vi "RT-test2.vi"(8 "布尔":bool, 9 "Load":bool, 10 "SimulatorConfig":T4, 11 "PatternConfig":T5 {"Max_Rate_[Hz]" format="%#_3p"}) -> (0 "EPTxPatternConfig":T1 {"Pattern"."Aux_4" format="%#_16g"; "Pattern"."Aux_3" format="%#_16g"; "Pattern"."Aux_2" format="%#_16g"; "Pattern"."Aux_1" format="%#_16g"; "Pattern"."Primary" format="%#_16g"}, 1 "Pattern Loading":bool, 2 "EPTxSimulatorConfig":T3, 3 "Sim Loading":bool, 4 "布尔 2":bool)   [LabVIEW 2020]
uses:
  <vilib>/Powertrain Controls/Device Drivers/Engine Position Tracking/EPTx/RevA/RT/Controls/Pattern Config.ctl
  <vilib>/Powertrain Controls/Device Drivers/Engine Position Tracking/EPTx/RevA/RT/Controls/Simulator Config.ctl
  <vilib>/Powertrain Controls/Device Drivers/Engine Position Tracking/EPTx/RevA/FPGA/Controls/EPTxSimulatorConfig.ctl
  <vilib>/Powertrain Controls/Device Drivers/Engine Position Tracking/EPTx/RevA/FPGA/Controls/EPTxPatternConfig.ctl
  <vilib>/Powertrain Controls/Device Drivers/Engine Position Tracking/EPTx/RevA/FPGA/Controls/Patterns.ctl
  <vilib>/Powertrain Controls/Device Drivers/Engine Position Tracking/EPTx/RevA/RT/Controls/EPTxPattern.ctl
  <vilib>/Powertrain Controls/Device Drivers/Engine Position Tracking/EPTx/RevA/RT/Controls/Pattern.ctl
  <vilib>/Powertrain Controls/Device Drivers/Engine Position Tracking/EPTx/RevA/RT/EPTx - RevA - RT.lvlib
  <vilib>/Powertrain Controls/Device Drivers/Engine Position Tracking/EPTx/RevA/FPGA/EPTx - RevA - FPGA.lvlib
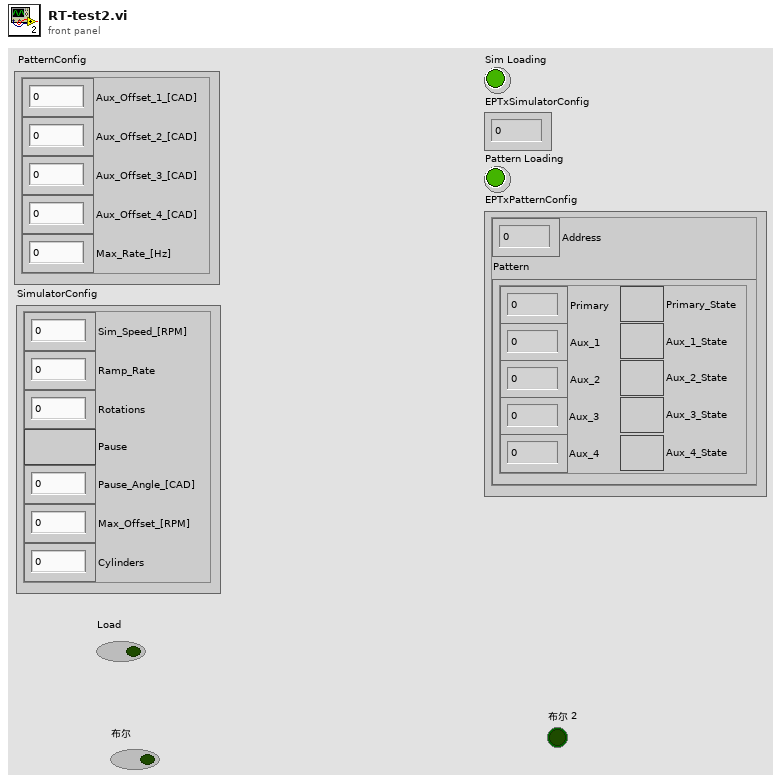
[diagram p1: front panel]
types:
  T1 = typedef "EPTx - RevA - FPGA.lvlib/EPTxPatternConfig.ctl" = cluster{"Address":fxp<+,14,14>, "Pattern":T2}
  T2 = typedef "EPTx - RevA - FPGA.lvlib/Patterns.ctl" = cluster{"Primary":fxp<+,19,12>, "Primary_State":bool, "Aux_1":fxp<+,19,12>, "Aux_1_State":bool, "Aux_2":fxp<+,19,12>, "Aux_2_State":bool, "Aux_3":fxp<+,19,12>, "Aux_3_State":bool, "Aux_4":fxp<+,19,12>, "Aux_4_State":bool}
  T3 = typedef "EPTx - RevA - FPGA.lvlib/EPTxSimulatorConfig.ctl" = u32
  T4 = typedef "EPTx - RevA - RT.lvlib/Simulator Config.ctl" = cluster{"Sim_Speed_[RPM]":sgl, "Ramp_Rate":sgl, "Rotations":u8, "Pause":bool, "Pause_Angle_[CAD]":sgl, "Max_Offset_[RPM]":sgl, "Cylinders":u8}
  T5 = typedef "EPTx - RevA - RT.lvlib/Pattern Config.ctl" = cluster{"Aux_Offset_1_[CAD]":sgl, "Aux_Offset_2_[CAD]":sgl, "Aux_Offset_3_[CAD]":sgl, "Aux_Offset_4_[CAD]":sgl, "Max_Rate_[Hz]":sgl}
  T6 = typedef "EPTx - RevA - RT.lvlib/EPTxPattern.ctl" = cluster{"Rotations":u8, "Cylinders":u8, "Primary":T7[], "Aux 1":T7[], "Aux 2":T7[], "Aux 3":T7[], "Aux 4":T7[]}
  T7 = typedef "EPTx - RevA - RT.lvlib/Pattern.ctl" = cluster{"Angle":sgl, "State":bool}
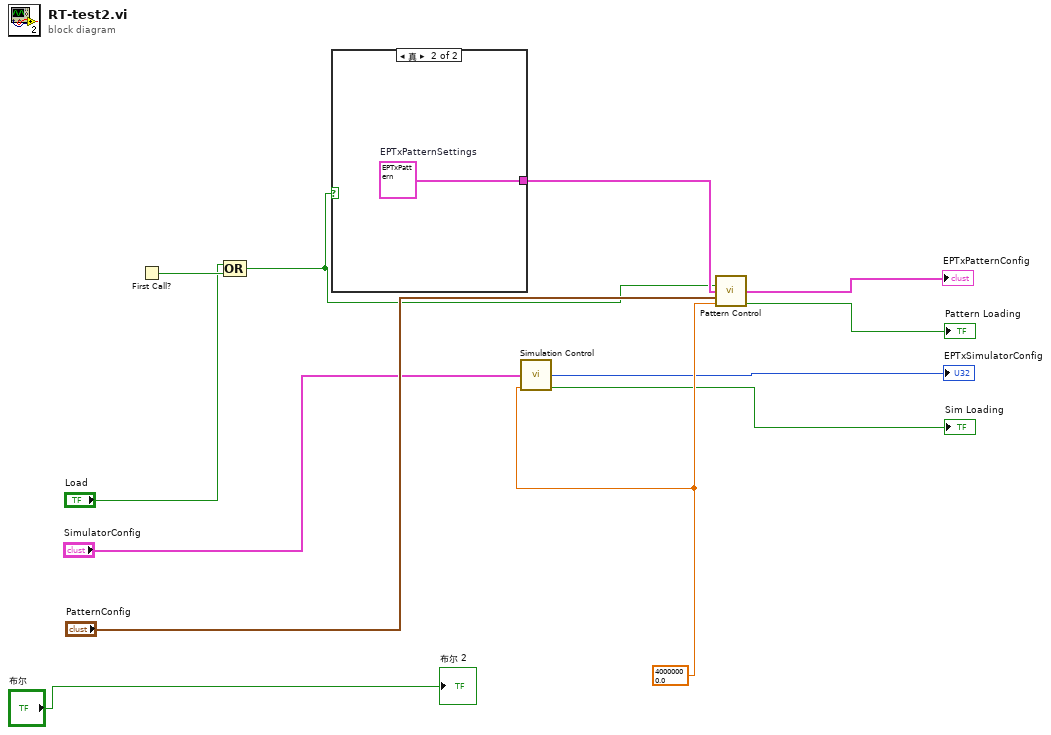
[diagram p0: block diagram]
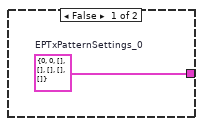
[diagram p2: hidden frame]
diagram:
  w9 = sgl 40000000.0 ("Frequency (40M) [Hz]")
  n1 = First Call?() -> (First Call?: T/F=w11:bool)
  n2 = Compound Arithmetic op=OR ("复合运算")("Load", w11) -> (w6:bool)
  n3 = case shown="真" w6 {
    tunnel: [w13 w14] -> w12
    frame False {
      w13 = T6 {"Rotations"=0, "Cylinders"=0, "Primary"=[], "Aux 1"=[], "Aux 2"=[], "Aux 3"=[], "Aux 4"=[]}  # EPTxPatternSettings_0
    }
    frame True {
      w14 = T6 {"Rotations"=2, "Cylinders"=6, "Primary"=[{"Angle"=0.0, "State"=FALSE}, {"Angle"=3.0, "State"=TRUE}, {"Angle"=6.0, "State"=FALSE}, {"Angle"=9.0, "State"=TRUE}, {"Angle"=12.0, "State"=FALSE}, {"Angle"=15.0, "State"=TRUE}, {"Angle"=18.0, "State"=FALSE}, {"Angle"=21.0, "State"=TRUE}, {"Angle"=24.0, "State"=FALSE}, {"Angle"=27.0, "State"=TRUE}, {"Angle"=30.0, "State"=FALSE}, {"Angle"=33.0, "State"=TRUE}, {"Angle"=36.0, "State"=FALSE}, {"Angle"=39.0, "State"=TRUE}, {"Angle"=42.0, "State"=FALSE}, {"Angle"=45.0, "State"=TRUE}, {"Angle"=48.0, "State"=FALSE}, {"Angle"=51.0, "State"=TRUE}, {"Angle"=54.0, "State"=FALSE}, {"Angle"=57.0, "State"=TRUE}, {"Angle"=60.0, "State"=FALSE}, {"Angle"=63.0, "State"=TRUE}, {"Angle"=66.0, "State"=FALSE}, {"Angle"=69.0, "State"=TRUE}, {"Angle"=72.0, "State"=FALSE}, {"Angle"=75.0, "State"=TRUE}, {"Angle"=78.0, "State"=FALSE}, {"Angle"=81.0, "State"=TRUE}, {"Angle"=84.0, "State"=FALSE}, {"Angle"=87.0, "State"=TRUE}, {"Angle"=90.0, "State"=FALSE}, {"Angle"=93.0, "State"=TRUE}, {"Angle"=96.0, "State"=FALSE}, {"Angle"=99.0, "State"=TRUE}, {"Angle"=102.0, "State"=FALSE}, {"Angle"=105.0, "State"=TRUE}, {"Angle"=108.0, "State"=FALSE}, {"Angle"=111.0, "State"=TRUE}, {"Angle"=114.0, "State"=FALSE}, {"Angle"=117.0, "State"=TRUE}, {"Angle"=120.0, "State"=FALSE}, {"Angle"=123.0, "State"=TRUE}, {"Angle"=126.0, "State"=FALSE}, {"Angle"=129.0, "State"=TRUE}, {"Angle"=132.0, "State"=FALSE}, {"Angle"=135.0, "State"=TRUE}, {"Angle"=138.0, "State"=FALSE}, {"Angle"=141.0, "State"=TRUE}, {"Angle"=144.0, "State"=FALSE}, {"Angle"=147.0, "State"=TRUE}, {"Angle"=150.0, "State"=FALSE}, {"Angle"=153.0, "State"=TRUE}, {"Angle"=156.0, "State"=FALSE}, {"Angle"=159.0, "State"=TRUE}, {"Angle"=162.0, "State"=FALSE}, {"Angle"=165.0, "State"=TRUE}, {"Angle"=168.0, "State"=FALSE}, {"Angle"=171.0, "State"=TRUE}, {"Angle"=174.0, "State"=FALSE}, {"Angle"=177.0, "State"=TRUE}, {"Angle"=180.0, "State"=FALSE}, {"Angle"=183.0, "State"=TRUE}, {"Angle"=186.0, "State"=FALSE}, {"Angle"=189.0, "State"=TRUE}, {"Angle"=192.0, "State"=FALSE}, {"Angle"=195.0, "State"=TRUE}, {"Angle"=198.0, "State"=FALSE}, {"Angle"=201.0, "State"=TRUE}, {"Angle"=204.0, "State"=FALSE}, {"Angle"=207.0, "State"=TRUE}, {"Angle"=210.0, "State"=FALSE}, {"Angle"=213.0, "State"=TRUE}, {"Angle"=216.0, "State"=FALSE}, {"Angle"=219.0, "State"=TRUE}, {"Angle"=222.0, "State"=FALSE}, {"Angle"=225.0, "State"=TRUE}, {"Angle"=228.0, "State"=FALSE}, {"Angle"=231.0, "State"=TRUE}, {"Angle"=234.0, "State"=FALSE}, {"Angle"=237.0, "State"=TRUE}, {"Angle"=240.0, "State"=FALSE}, {"Angle"=243.0, "State"=TRUE}, {"Angle"=246.0, "State"=FALSE}, {"Angle"=249.0, "State"=TRUE}, {"Angle"=252.0, "State"=FALSE}, {"Angle"=255.0, "State"=TRUE}, {"Angle"=258.0, "State"=FALSE}, {"Angle"=261.0, "State"=TRUE}, {"Angle"=264.0, "State"=FALSE}, {"Angle"=267.0, "State"=TRUE}, {"Angle"=270.0, "State"=FALSE}, {"Angle"=273.0, "State"=TRUE}, {"Angle"=276.0, "State"=FALSE}, {"Angle"=279.0, "State"=TRUE}, {"Angle"=282.0, "State"=FALSE}, {"Angle"=285.0, "State"=TRUE}, {"Angle"=288.0, "State"=FALSE}, {"Angle"=291.0, "State"=TRUE}, {"Angle"=294.0, "State"=FALSE}, {"Angle"=297.0, "State"=TRUE}, {"Angle"=300.0, "State"=FALSE}, {"Angle"=303.0, "State"=TRUE}, {"Angle"=306.0, "State"=FALSE}, {"Angle"=309.0, "State"=TRUE}, {"Angle"=312.0, "State"=FALSE}, {"Angle"=315.0, "State"=TRUE}, {"Angle"=318.0, "State"=FALSE}, {"Angle"=321.0, "State"=TRUE}, {"Angle"=324.0, "State"=FALSE}, {"Angle"=327.0, "State"=TRUE}, {"Angle"=330.0, "State"=FALSE}, {"Angle"=333.0, "State"=TRUE}, {"Angle"=336.0, "State"=FALSE}, {"Angle"=339.0, "State"=TRUE}, {"Angle"=342.0, "State"=FALSE}, {"Angle"=345.0, "State"=TRUE}, {"Angle"=360.0, "State"=FALSE}, {"Angle"=363.0, "State"=TRUE}, {"Angle"=366.0, "State"=FALSE}, {"Angle"=369.0, "State"=TRUE}, {"Angle"=372.0, "State"=FALSE}, {"Angle"=375.0, "State"=TRUE}, {"Angle"=378.0, "State"=FALSE}, {"Angle"=381.0, "State"=TRUE}, {"Angle"=384.0, "State"=FALSE}, {"Angle"=387.0, "State"=TRUE}, {"Angle"=390.0, "State"=FALSE}, {"Angle"=393.0, "State"=TRUE}, {"Angle"=396.0, "State"=FALSE}, {"Angle"=399.0, "State"=TRUE}, {"Angle"=402.0, "State"=FALSE}, {"Angle"=405.0, "State"=TRUE}, {"Angle"=408.0, "State"=FALSE}, {"Angle"=411.0, "State"=TRUE}, {"Angle"=414.0, "State"=FALSE}, {"Angle"=417.0, "State"=TRUE}, {"Angle"=420.0, "State"=FALSE}, {"Angle"=423.0, "State"=TRUE}, {"Angle"=426.0, "State"=FALSE}, {"Angle"=429.0, "State"=TRUE}, {"Angle"=432.0, "State"=FALSE}, {"Angle"=435.0, "State"=TRUE}, {"Angle"=438.0, "State"=FALSE}, {"Angle"=441.0, "State"=TRUE}, {"Angle"=444.0, "State"=FALSE}, {"Angle"=447.0, "State"=TRUE}, {"Angle"=450.0, "State"=FALSE}, {"Angle"=453.0, "State"=TRUE}, {"Angle"=456.0, "State"=FALSE}, {"Angle"=459.0, "State"=TRUE}, {"Angle"=462.0, "State"=FALSE}, {"Angle"=465.0, "State"=TRUE}, {"Angle"=468.0, "State"=FALSE}, {"Angle"=471.0, "State"=TRUE}, {"Angle"=474.0, "State"=FALSE}, {"Angle"=477.0, "State"=TRUE}, {"Angle"=480.0, "State"=FALSE}, {"Angle"=483.0, "State"=TRUE}, {"Angle"=486.0, "State"=FALSE}, {"Angle"=489.0, "State"=TRUE}, {"Angle"=492.0, "State"=FALSE}, {"Angle"=495.0, "State"=TRUE}, {"Angle"=498.0, "State"=FALSE}, {"Angle"=501.0, "State"=TRUE}, {"Angle"=504.0, "State"=FALSE}, {"Angle"=507.0, "State"=TRUE}, {"Angle"=510.0, "State"=FALSE}, {"Angle"=513.0, "State"=TRUE}, {"Angle"=516.0, "State"=FALSE}, {"Angle"=519.0, "State"=TRUE}, {"Angle"=522.0, "State"=FALSE}, {"Angle"=525.0, "State"=TRUE}, {"Angle"=528.0, "State"=FALSE}, {"Angle"=531.0, "State"=TRUE}, {"Angle"=534.0, "State"=FALSE}, {"Angle"=537.0, "State"=TRUE}, {"Angle"=540.0, "State"=FALSE}, {"Angle"=543.0, "State"=TRUE}, {"Angle"=546.0, "State"=FALSE}, {"Angle"=549.0, "State"=TRUE}, {"Angle"=552.0, "State"=FALSE}, {"Angle"=555.0, "State"=TRUE}, {"Angle"=558.0, "State"=FALSE}, {"Angle"=561.0, "State"=TRUE}, {"Angle"=564.0, "State"=FALSE}, {"Angle"=567.0, "State"=TRUE}, {"Angle"=570.0, "State"=FALSE}, {"Angle"=573.0, "State"=TRUE}, {"Angle"=576.0, "State"=FALSE}, {"Angle"=579.0, "State"=TRUE}, {"Angle"=582.0, "State"=FALSE}, {"Angle"=585.0, "State"=TRUE}, {"Angle"=588.0, "State"=FALSE}, {"Angle"=591.0, "State"=TRUE}, {"Angle"=594.0, "State"=FALSE}, {"Angle"=597.0, "State"=TRUE}, {"Angle"=600.0, "State"=FALSE}, {"Angle"=603.0, "State"=TRUE}, {"Angle"=606.0, "State"=FALSE}, {"Angle"=609.0, "State"=TRUE}, {"Angle"=612.0, "State"=FALSE}, {"Angle"=615.0, "State"=TRUE}, {"Angle"=618.0, "State"=FALSE}, {"Angle"=621.0, "State"=TRUE}, {"Angle"=624.0, "State"=FALSE}, {"Angle"=627.0, "State"=TRUE}, {"Angle"=630.0, "State"=FALSE}, {"Angle"=633.0, "State"=TRUE}, {"Angle"=636.0, "State"=FALSE}, {"Angle"=639.0, "State"=TRUE}, {"Angle"=642.0, "State"=FALSE}, {"Angle"=645.0, "State"=TRUE}, {"Angle"=648.0, "State"=FALSE}, {"Angle"=651.0, "State"=TRUE}, {"Angle"=654.0, "State"=FALSE}, {"Angle"=657.0, "State"=TRUE}, {"Angle"=660.0, "State"=FALSE}, {"Angle"=663.0, "State"=TRUE}, {"Angle"=666.0, "State"=FALSE}, {"Angle"=669.0, "State"=TRUE}, {"Angle"=672.0, "State"=FALSE}, {"Angle"=675.0, "State"=TRUE}, {"Angle"=678.0, "State"=FALSE}, {"Angle"=681.0, "State"=TRUE}, {"Angle"=684.0, "State"=FALSE}, {"Angle"=687.0, "State"=TRUE}, {"Angle"=690.0, "State"=FALSE}, {"Angle"=693.0, "State"=TRUE}, {"Angle"=696.0, "State"=FALSE}, {"Angle"=699.0, "State"=TRUE}, {"Angle"=702.0, "State"=FALSE}, {"Angle"=705.0, "State"=TRUE}], "Aux 1"=[{"Angle"=12.0, "State"=TRUE}, {"Angle"=24.0, "State"=FALSE}, {"Angle"=48.0, "State"=TRUE}, {"Angle"=60.0, "State"=FALSE}, {"Angle"=132.0, "State"=TRUE}, {"Angle"=144.0, "State"=FALSE}, {"Angle"=198.0, "State"=TRUE}, {"Angle"=252.0, "State"=TRUE}, {"Angle"=264.0, "State"=FALSE}, {"Angle"=318.0, "State"=TRUE}, {"Angle"=372.0, "State"=TRUE}, {"Angle"=384.0, "State"=FALSE}, {"Angle"=438.0, "State"=TRUE}, {"Angle"=492.0, "State"=TRUE}, {"Angle"=504.0, "State"=FALSE}, {"Angle"=558.0, "State"=TRUE}, {"Angle"=612.0, "State"=TRUE}, {"Angle"=624.0, "State"=FALSE}, {"Angle"=678.0, "State"=TRUE}], "Aux 2"=[{"Angle"=12.0, "State"=TRUE}, {"Angle"=24.0, "State"=FALSE}, {"Angle"=48.0, "State"=TRUE}, {"Angle"=60.0, "State"=FALSE}, {"Angle"=132.0, "State"=TRUE}, {"Angle"=144.0, "State"=FALSE}, {"Angle"=198.0, "State"=TRUE}, {"Angle"=252.0, "State"=TRUE}, {"Angle"=264.0, "State"=FALSE}, {"Angle"=318.0, "State"=TRUE}, {"Angle"=372.0, "State"=TRUE}, {"Angle"=384.0, "State"=FALSE}, {"Angle"=438.0, "State"=TRUE}, {"Angle"=492.0, "State"=TRUE}, {"Angle"=504.0, "State"=FALSE}, {"Angle"=558.0, "State"=TRUE}, {"Angle"=612.0, "State"=TRUE}, {"Angle"=624.0, "State"=FALSE}, {"Angle"=678.0, "State"=TRUE}], "Aux 3"=[], "Aux 4"=[]}  # EPTxPatternSettings
    }
  }
  n4 = call <vilib>:"Simulation Control.vi"("SimulatorConfig"="SimulatorConfig", "Frequency (40M) [Hz]"=w9) -> ("EPTxSimulatorConfig"=→"EPTxSimulatorConfig":T3, "Loading"=→"Sim Loading":bool)  [unwired: 12 in]
  n5 = call <vilib>:"Pattern Control.vi"("Load"=w6, "EPTxPatternSettings"=w12, "PatternConfig"="PatternConfig", "Frequency (40M) [Hz]"=w9) -> ("EPTxPatternConfig"=→"EPTxPatternConfig":T1, "Loading"=→"Pattern Loading":bool)  [unwired: 10 in]
  "布尔 2" <- "布尔"
